vi "Lookup APIs of Type.vi"(8 "error in (no error)":errorcluster, 10 "Identity - Type Only":refnum<class "Identity.lvclass">, 11 "VolatusAPI in":refnum<class "VolatusAPI.lvclass">) -> (0 "error out":errorcluster, 2 "APIs":refnum<class "API.lvclass">[](array[class]), 3 "VolatusAPI out":refnum<class "VolatusAPI.lvclass">)   [LabVIEW 2020, in "Volatus.lvlib" / "VolatusAPI.lvclass"]
uses:
  VolatusAPI.lvclass
  VolatusAPI.lvclass/VolatusAPI.ctl
  VolatusCore Messages/Lookup APIs of Type Msg/Lookup APIs of Type Msg.lvclass
  lv-promises/Promises/Promise/Promise.lvclass
  ApiArrayValue/ApiArrayValue.lvclass
  lv-promises/Promises/Future/Future.lvclass
  C:/dev/lv20CE/relink/lv-promises/Promises/Value/Value.lvclass
  C:/dev/lv20CE/relink/lv-volatus/Volatus/ApiArrayValue/ApiArrayValue.lvclass
  Identity/Identity.lvclass
  API/API.lvclass
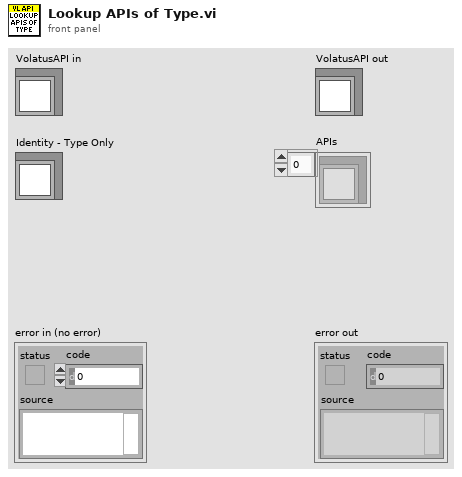
[diagram p1: front panel]
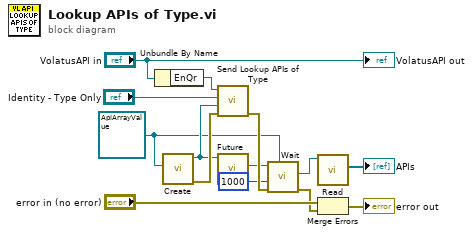
[diagram p0: block diagram]
diagram:
  w5 = refnum<class "ApiArrayValue.lvclass"> refnum ("Volatus:ApiArrayValue.lvclass")
  n1 = Unbundle By Name("VolatusAPI in") -> ("EnQr"=w11:refnum<class "Message Enqueuer.lvclass">)
  n2 = call "Create.vi"("Result Type"=w5) -> ("error out"=w9:errorcluster, "Promise"=w8:refnum<class "Promise.lvclass">)  [unwired: 9 in]
  n3 = call "Send Lookup APIs of Type.vi"("error in (no error)"=w9, "Futures:Promise"=w8, "Identity - Type Only"="Identity - Type Only", "Message Enqueuer"=w11) -> ("error out"=w14:errorcluster)  [unwired: 6 in, 1 out]
  n4 = call "Future.vi"("Promise in"=w8) -> ("Future"=w7:refnum<class "Future.lvclass">)  [unwired: 9 in, 1 out]
  n5 = call "Wait.vi"("Result Type"=w5, "error in (no error)"=w14, "Timeout mS (-1)"=1000, "Future in"=w7) -> ("error out"=w1:errorcluster, "Result"=w4:refnum<class "ApiArrayValue.lvclass">)  [unwired: 6 in]
  n6 = call "Read.vi"("ApiArrayValue in"=w4) -> ("APIs"=→"APIs":refnum<class "API.lvclass">[])  [unwired: 10 in]
  n7 = Merge Errors("error in (no error)", w1) -> (→"error out":errorcluster)
  "VolatusAPI out" <- "VolatusAPI in"
